vi "array_formula.vi"() -> ()   [LabVIEW 8.6]
panel:
  out "error out":errorcluster
  out "function return 2":string
  # "array_formula.xlsx"
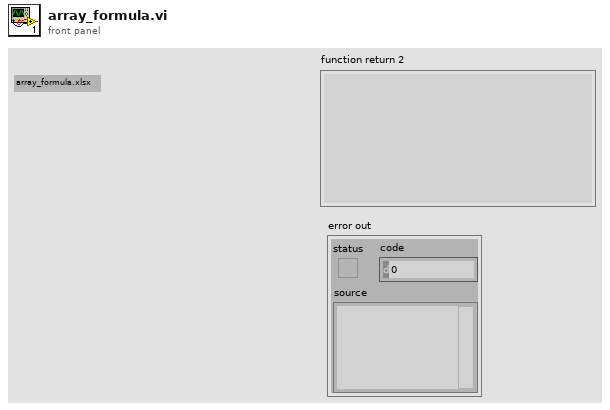
[diagram p1: front panel]
types:
  T1 = enum32{"invalid app kind", "Development System", "Run Time System", "Student Edition", "Embedded LabVIEW", "Evaluation", "Custom"}
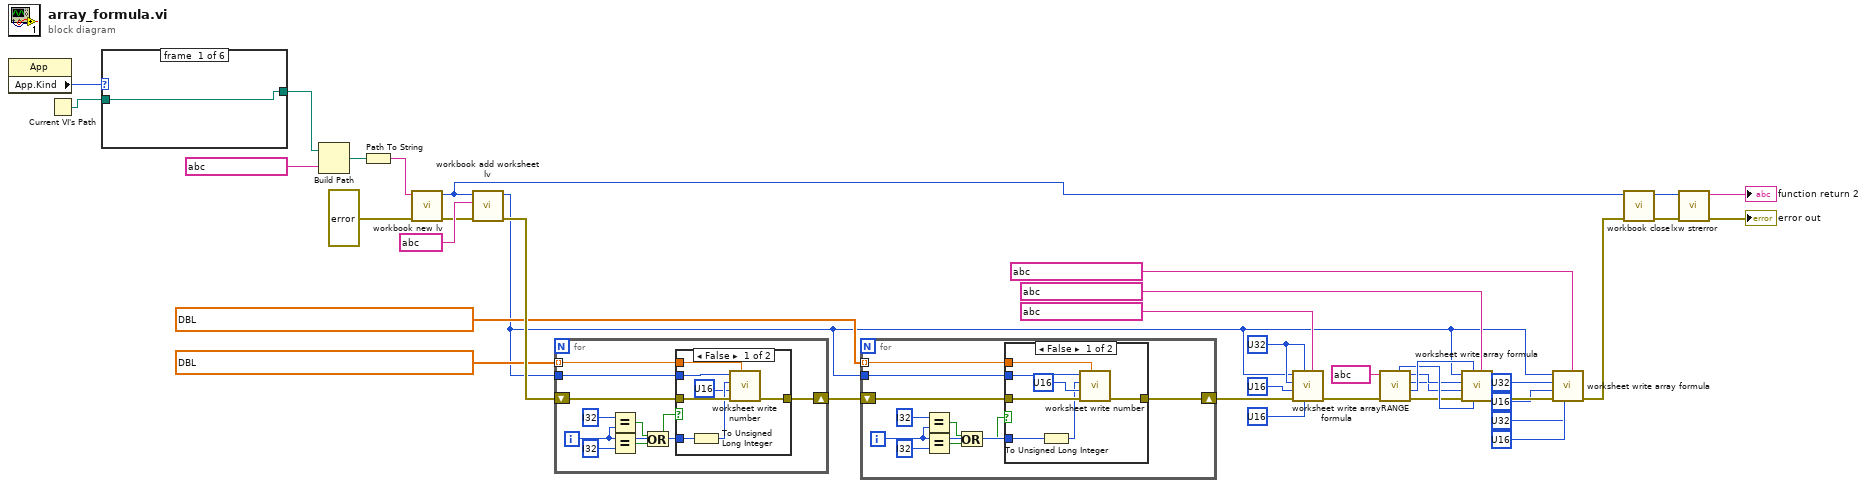
[diagram p0: block diagram]
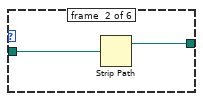
[diagram p4: hidden frame]
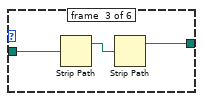
[diagram p5: hidden frame]
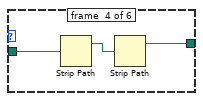
[diagram p6: hidden frame]
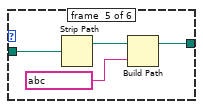
[diagram p7: hidden frame]
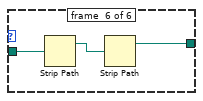
[diagram p8: hidden frame]
diagram:
  w19 = u32 ? ("last_row")
  n1 = property class="App"() -> ("App.Kind"=w39:T1)  [unwired: 2 in, 2 out]
  n2 = Current VI's Path() -> (path=w38:path)
  n3 = case shown="\"Evaluation\"" w39 {
    tunnel: w38 -> [w40 w42 w45 w48 w52 w55]
    tunnel: [w40 w41 w43 w46 w50 w53] -> w37
    frame #0 {
    }
    frame #1 {
      n4 = Strip Path(path=w42) -> (stripped path=w41:path)  [unwired: 1 out]
    }
    frame #2 {
      n5 = Strip Path(path=w45) -> (stripped path=w44:path)  [unwired: 1 out]
      n6 = Strip Path(path=w44) -> (stripped path=w43:path)  [unwired: 1 out]
    }
    frame #3 {
      n7 = Strip Path(path=w48) -> (stripped path=w47:path)  [unwired: 1 out]
      n8 = Strip Path(path=w47) -> (stripped path=w46:path)  [unwired: 1 out]
    }
    frame #4 {
      n9 = Strip Path(path=w52) -> (stripped path=w51:path)  [unwired: 1 out]
      n10 = Build Path(base path=w51, name or relative path=string ?) -> (appended path=w50:path)
    }
    frame #5 {
      n11 = Strip Path(path=w55) -> (stripped path=w54:path)  [unwired: 1 out]
      n12 = Strip Path(path=w54) -> (stripped path=w53:path)  [unwired: 1 out]
    }
  }
  n13 = Build Path(base path=w37, name or relative path=string ? ("filename")) -> (appended path=w27:path)
  n14 = Path To String(path=w27) -> (string=w26:string)
  n15 = call "workbook new lv.vi"("error in (no error)"=errorcluster ?, "filename"=w26) -> ("error out"=w34:errorcluster, "function return"=w28:u32)  [unwired: 8 in]
  n16 = call "workbook add worksheet lv.vi"("error in (no error)"=w34, "sheetname"=string ?, "workbook"=w28) -> ("error out"=w25:errorcluster, "function return"=w5:u32)  [unwired: 7 in]
  n17 = for {
    tunnel: dbl[] ? -> [w64] mode=indexing
    tunnel: w5 -> [w63]
    shift-right: [w62] -> w23
    shift-left: w25 -> [w65]
    i -> [w56]
    n18 = Equal?(x=i32 ?, y=w56) -> (x = y?=w60:bool)
    n19 = Equal?(x=w56, y=i32 ?) -> (x = y?=w61:bool)
    n20 = Or(x=w60, y=w61) -> (x .or. y?=w57:bool)
    n21 = case shown="False" w57 {
      tunnel: w65 -> [w72 w73]
      tunnel: w64 -> [w71 _]
      tunnel: w63 -> [w70 _]
      tunnel: w56 -> [w69 _]
      tunnel: [w67 w73] -> w62
      frame #0 {
        n22 = To Unsigned Long Integer(number=w69) -> (unsigned 32bit integer=w68:u32)
        n23 = call "worksheet write number.vi"("number"=w71, "error in (no error)"=w72, "col"=u16 ?, "row"=w68, "worksheet"=w70) -> ("error out"=w67:errorcluster)  [unwired: 5 in, 1 out]
      }
      frame #1 {
      }
    }
  }
  n24 = for {
    tunnel: dbl[] ? -> [w82] mode=indexing
    tunnel: w5 -> [w81]
    shift-right: [w80] -> w21
    shift-left: w23 -> [w83]
    i -> [w75]
    n25 = Equal?(x=i32 ?, y=w75) -> (x = y?=w78:bool)
    n26 = Equal?(x=w75, y=i32 ?) -> (x = y?=w79:bool)
    n27 = Or(x=w78, y=w79) -> (x .or. y?=w74:bool)
    n28 = case shown="False" w74 {
      tunnel: w83 -> [w90 w91]
      tunnel: w82 -> [w89 _]
      tunnel: w81 -> [w88 _]
      tunnel: w75 -> [w86 _]
      tunnel: [w84 w91] -> w80
      frame #0 {
        n29 = To Unsigned Long Integer(number=w86) -> (unsigned 32bit integer=w85:u32)
        n30 = call "worksheet write number.vi"("number"=w89, "error in (no error)"=w90, "col"=u16 ?, "row"=w85, "worksheet"=w88) -> ("error out"=w84:errorcluster)  [unwired: 5 in, 1 out]
      }
      frame #1 {
      }
    }
  }
  n31 = call "worksheet write array formula.vi"("formula"=string ?, "last_col"=u16 ?, "last_row"=w19, "error in (no error)"=w21, "first_col"=u16 ?, "first_row"=w19, "worksheet"=w5) -> ("error out"=w9:errorcluster)  [unwired: 3 in, 1 out]
  n32 = call "RANGE.vi"("error in (no error)"=w9, "range_str"=string ?) -> ("error out"=w10:errorcluster, "row2"=w14:u32, "col"=w11:u16, "row"=w12:u32, "col2"=w13:u16)  [unwired: 5 in]
  n33 = call "worksheet write array formula.vi"("formula"=string ?, "last_col"=w13, "last_row"=w14, "error in (no error)"=w10, "first_col"=w11, "first_row"=w12, "worksheet"=w5) -> ("error out"=w16:errorcluster)  [unwired: 3 in, 1 out]
  n34 = call "worksheet write array formula.vi"("formula"=string ?, "last_col"=u16 ?, "last_row"=u32 ?, "error in (no error)"=w16, "first_col"=u16 ?, "first_row"=u32 ?, "worksheet"=w5) -> ("error out"=w15:errorcluster)  [unwired: 3 in, 1 out]
  n35 = call "workbook close.vi"("error in (no error)"=w15, "workbook"=w28) -> ("error out"=w30:errorcluster, "function return"=w32:u32)  [unwired: 8 in]
  n36 = call "lxw strerror.vi"("error in (no error)"=w30, "error_num"=w32) -> ("error out"=→"error out":errorcluster, "function return"=→"function return 2":string)  [unwired: 8 in]
